vi "sendToFPGA.vi"(8 "error in (no error)":errorcluster, 10 "Data":u16[](array[numeric]), 11 "ModbusPort1 in":refnum<class "ModbusPort3.lvclass">) -> (0 "error out":errorcluster, 3 "ModbusPort1 out":refnum<class "ModbusPort3.lvclass">)   [LabVIEW 2015, in "ModbusPort3.lvclass"]
uses:
  ModbusPort3.lvclass
  Modbus/Modbus.lvclass/Modbus.ctl
  <vilib>/Utility/error.llb/Error Cluster From Error Code.vi
  <vilib>/rvi/errors/niLvFpgaAdjustHostInterfaceError.vi
  <vilib>/rvi/interface/nirviMethod/nirviMethod.xnode
  Modbus/Modbus.lvclass
  <vilib>/FPGAPlugInAG/Dynamic/niLvFpga_WriteFifo_Dynamic.vi
  <vilib>/rvi/errors/niLvFpgaMergeErrorWithErrorCode.vi
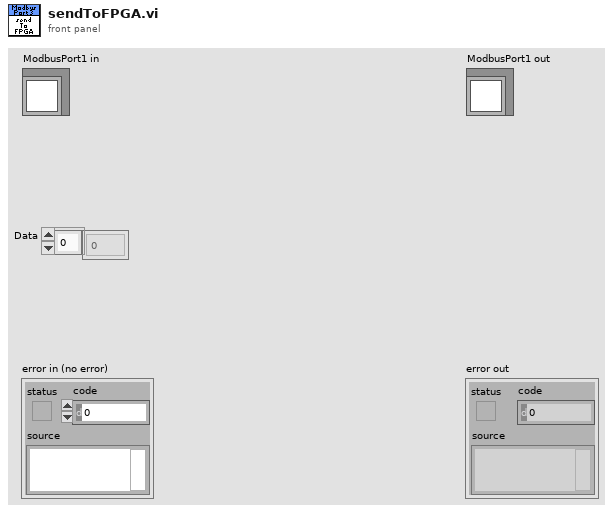
[diagram p1: front panel]
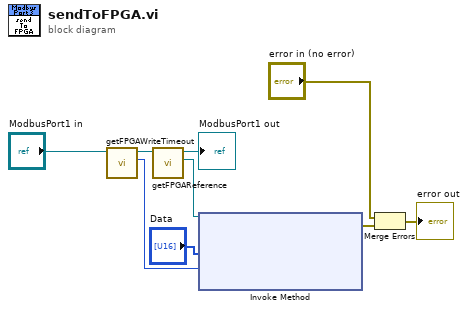
[diagram p0: block diagram]
diagram:
  n1 = call "getFPGAWriteTimeout.vi"("Modbus in"="ModbusPort1 in") -> ("FPGAWriteTimeout"=w6:i32, "Modbus out"=w7:refnum<class "ModbusPort3.lvclass">)  [unwired: 9 in]
  n2 = call "getFPGAReference.vi"("Modbus in"=w7) -> ("FPGAReference"=w9:refnum<k20>, "Modbus out"=→"ModbusPort1 out":refnum<class "ModbusPort3.lvclass">)  [unwired: 9 in]
  n3 = xnode "Invoke Method"("FPGA VI Reference In"=w9, "Data"="Data", "Timeout (ms)"=w6) -> ("error out"=w5:errorcluster)  [unwired: 1 in, 2 out]
  n4 = Merge Errors("error in (no error)", w5) -> (→"error out":errorcluster)
